vi "Get LVObject.vi"(8 "error in (no error)":errorcluster, 9 "Object Type":refnum<class>, 10 "Offset":i32, 11 "JSON String containing Flattened Object":string) -> (0 "error out":errorcluster, 1 "Object out":refnum<class>, 2 "Offset past match":i32)   [LabVIEW 2020, in "JSONtext.lvlib"]
doc: "Gets LabVIEW Object that has been flattened and stored as a JSON String."
uses:
  <vilib>/JDP Science/JSONtext/JSONtext.lvlib
  <vilib>/JDP Science/JSONtext/Parsing/Advance past String.vi
  <vilib>/JDP Science/JSONtext/String Subset.vi
  <vilib>/JDP Science/JSONtext/support/Strip Quotes and Unescape.vi
  <vilib>/JDP Science/JSONtext/support/Unescape JSON string.vi
  <vilib>/JDP Science/JSONtext/Parsing/Parsing Error in converting to LabVIEW type.vi
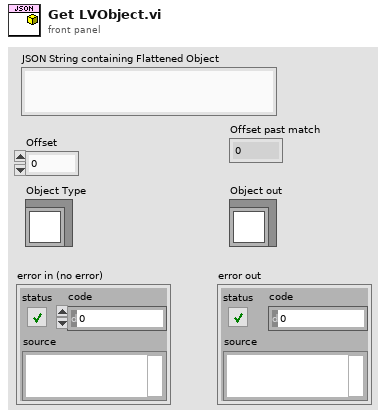
[diagram p1: front panel]
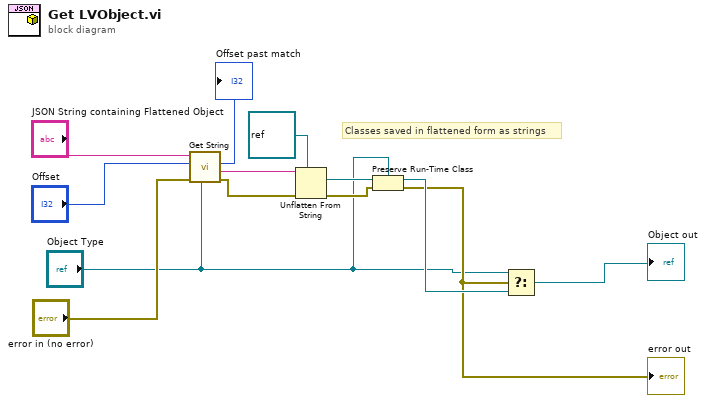
[diagram p0: block diagram]
diagram:
  # "Classes saved in flattened form as strings"
  n1 = call <vilib>:"Get String.vi"("LV Type"="Object Type", "error in (no error)"="error in (no error)", "Offset"="Offset", "JSON"="JSON String containing Flattened Object") -> ("error out"=w12:errorcluster, "String"=w6:string, "Offset past match"=→"Offset past match":i32)  [unwired: 5 in]
  n2 = Unflatten From String(type=refnum<class> refnum ("LabVIEW Object"), binary string=w6, error in (no error)=w12) -> (value=w7:refnum<class>, error out=w8:errorcluster)  [unwired: 2 in, 1 out]
  n3 = Preserve Run-Time Class(object in=w7, error in=w8, 2:"Object Type") -> (object out=w10:refnum<class>, error out=w9:errorcluster)
  "error out" <- w9
  n4 = Select(t="Object Type", s=w9, f=w10) -> (s? t:f=→"Object out":refnum<class>)
